vi "check_everything2.vi"(0 "VISA引用句柄输入":refnum<visa-resource-name>, 1 "数值输入":i32, 5 "错误输入（无错误）":errorcluster) -> (6 "电流值回读":string, 7 "键盘锁":string="CC", 8 "电压设置回读":string, 9 "过压设置值回读":string, 10 "过温":string, 11 "电流设置回读":string, 12 "数值输出":i32, 13 "电压值回读":string, 14 "CC/CV":string, 15 "蜂鸣器":string, 16 "测量模式":string, 17 "过压":string, 18 "On/Off":string, 19 "错误输出":errorcluster)   [LabVIEW 2012]
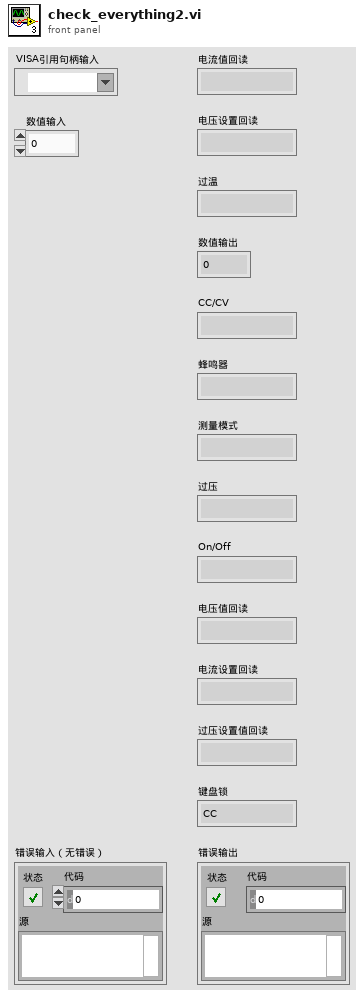
[diagram p1: front panel]
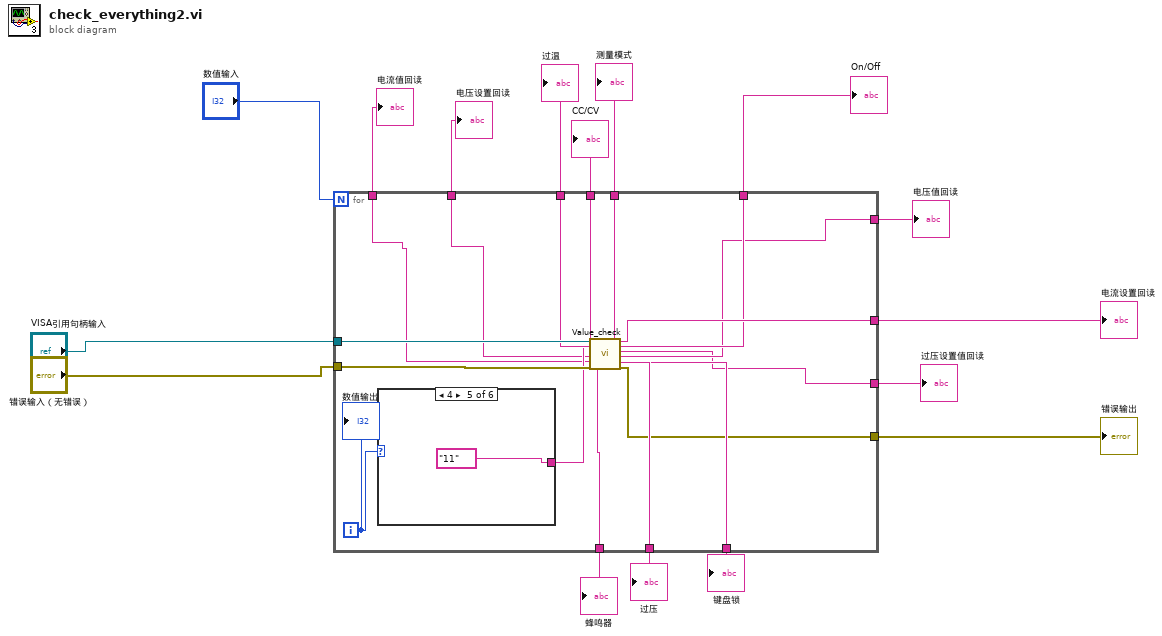
[diagram p0: block diagram]
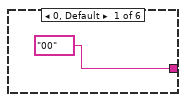
[diagram p2: hidden frame]
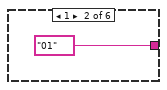
[diagram p3: hidden frame]
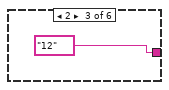
[diagram p4: hidden frame]
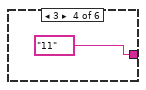
[diagram p5: hidden frame]
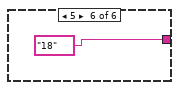
[diagram p6: hidden frame]
diagram:
  n1 = for {
    N: "数值输入" -> [_]
    tunnel: "VISA引用句柄输入" -> [w33]
    tunnel: "错误输入（无错误）" -> [w32]
    tunnel: [w31] -> w15
    tunnel: [w30] -> w3
    tunnel: [w29] -> w4
    tunnel: [w28] -> w5
    tunnel: [w27] -> w6
    tunnel: [w26] -> w7
    tunnel: [w25] -> w8
    tunnel: [w24] -> w9
    tunnel: [w21] -> w11
    tunnel: [w20] -> w12
    tunnel: [w19] -> w13
    tunnel: [w18] -> w14
    tunnel: [w17] -> w16
    i -> [w22]
    n2 = case shown="4" w22 {
      tunnel: ["00" "01" "12" "11" "11" "18"] -> w23
      frame 0, Default {
      }
      frame 1 {
      }
      frame 2 {
      }
      frame 3 {
      }
      frame 4 {
      }
      frame 5 {
      }
    }
    n3 = call "Value_check.vi"("VISA引用句柄输入"=w33, "Status Code"=w23, "错误输入（无错误）"=w32) -> ("电压设置回读"=w20:string, "电流值回读"=w21:string, "过温"=w29:string, "蜂鸣器"=w26:string, "测量模式"=w28:string, "过压"=w25:string, "CC/CV"=w27:string, "键盘锁"=w24:string, "电流设置回读"=w31:string, "On/Off"=w30:string, "过压设置值回读"=w18:string, "电压值回读"=w19:string, "错误输出"=w17:errorcluster)  [unwired: 3 in, 1 out]
    "数值输出" <- w22
  }
  "键盘锁" <- w9
  "错误输出" <- w16
  "电流设置回读" <- w15
  "过压设置值回读" <- w14
  "电压值回读" <- w13
  "电压设置回读" <- w12
  "电流值回读" <- w11
  "过压" <- w8
  "蜂鸣器" <- w7
  "CC/CV" <- w6
  "测量模式" <- w5
  "过温" <- w4
  "On/Off" <- w3
